vi "Global1.vi"() -> ()   [LabVIEW 2019]
panel:
  out "Button 5":bool
  out "Button 4":bool
  out "Button 3":bool
  out "Button 2":bool
  out "Axe 5":dbl
  out "Axe 4":dbl
  out "Axe 3":dbl
  out "Axe 2":dbl
  out "Axe 1":dbl
  out "Axe 0":dbl
  out "TestOutput":dbl
  out "Button 0":bool
  out "Button 1":bool
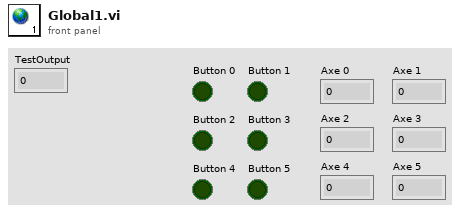
[diagram p1: front panel]
diagram:
